vi "Convert RGB to HSL.vi"(11 "Color Box":u32(colorbox)=16777215) -> (1 "L (%)":dbl, 2 "S (%)":dbl, 3 "H (deg)":dbl format="%#_2p")   [LabVIEW 2015, in "ColorSelector.lvclass"]
doc: "This VI will convert the RGB Color Scale to the HSL Color Scale.\n<b> </b> <b> </b>\n©2017 Q Software Innovations, LLC (QSI)\nwritten by Quentin Alldredge\nproduced in LabVIEW 2015\n\nsupport@qsoftwareinnovations.com\nwww.qsoftwareinnovations.com\n\nAll rights reserved.\n\nRedistribution and use in source and binary forms, with or without modification, are permitted provided that the following conditions are met:\n\n * Redistributions of source code must retain the above copyright notice, this list of conditions and the following disclaimer.\n * Redistributions in binary form must reproduce the above copyright notice, this list of conditions and the following disclaimer in the documentation and/or other materials provided with the distribution.\n * Neither the name of Q Software Innovations, LLC. nor the names of its contributors may be used to endorse or promote products derived from this software without specific prior written permission.\n\nTHIS SOFTWARE IS PROVIDED BY THE COPYRIGHT HOLDERS AND CONTRIBUTORS \"AS IS\" AND ANY EXPRESS OR IMPLIED WARRANTIES, INCLUDING, BUT NOT LIMITED TO, THE IMPLIED WARRANTIES OF MERCHANTABILITY AND FITNESS FOR A PARTICULAR PURPOSE ARE DISCLAIMED. IN NO EVENT SHALL THE COPYRIGHT OWNER OR CONTRIBUTORS BE LIABLE FOR ANY DIRECT, INDIRECT, INCIDENTAL, SPECIAL, EXEMPLARY, OR CONSEQUENTIAL DAMAGES (INCLUDING, BUT NOT LIMITED TO, PROCUREMENT OF SUBSTITUTE GOODS OR SERVICES; LOSS OF USE, DATA, OR PROFITS; OR BUSINESS INTERRUPTION) HOWEVER CAUSED AND ON ANY THEORY OF LIABILITY, WHETHER IN CONTRACT, STRICT LIABILITY, OR TORT (INCLUDING NEGLIGENCE OR OTHERWISE) ARISING IN ANY WAY OUT OF THE USE OF THIS SOFTWARE, EVEN IF ADVISED OF THE POSSIBILITY OF SUCH DAMAGE."
uses:
  ColorSelector.lvclass
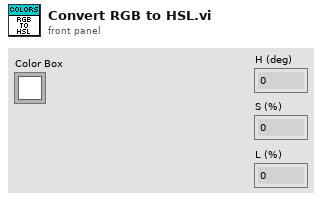
[diagram p1: front panel]
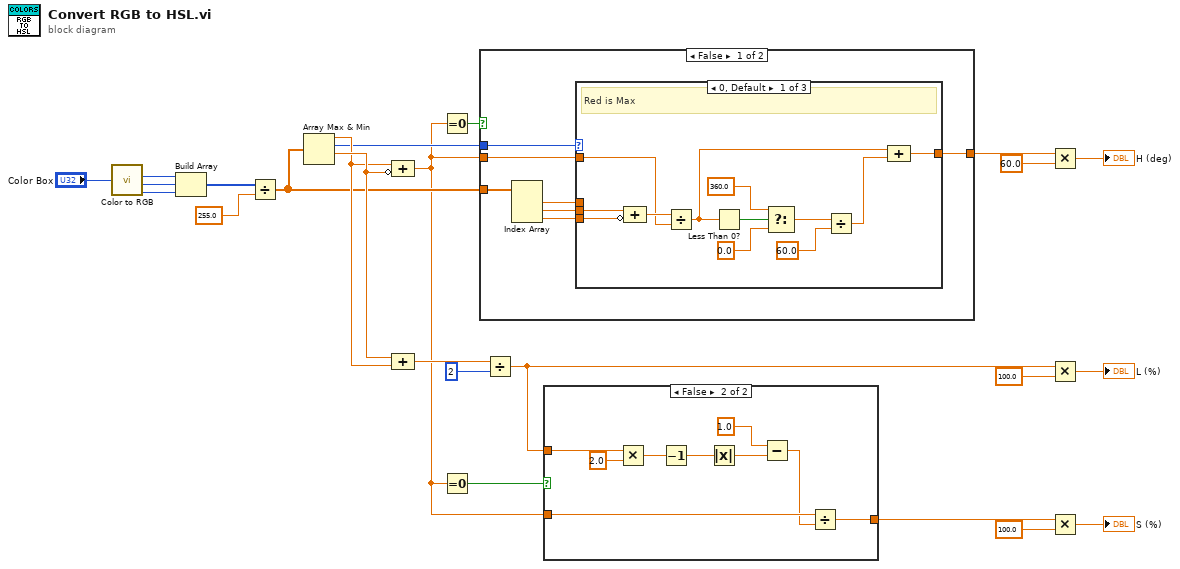
[diagram p0: block diagram]
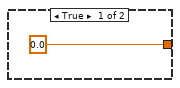
[diagram p2: hidden frame]
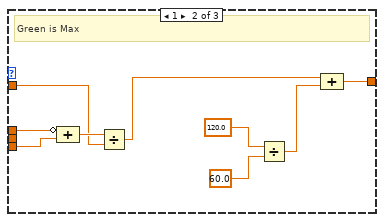
[diagram p3: hidden frame]
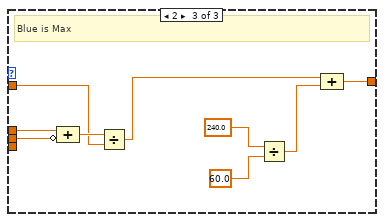
[diagram p4: hidden frame]
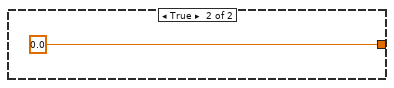
[diagram p5: hidden frame]
diagram:
  n1 = call <vilib>:"Color to RGB.vi"("Color"="Color Box") -> ("R"=w5:u8, "G"=w4:u8, "B"=w3:u8)  [unwired: 1 out]
  n2 = Build Array(w5, w4, w3) -> (w17:u8[])
  n3 = Divide(x=w17, y=255.0 ("x")) -> (x/y=w15:dbl[])
  n4 = Array Max & Min(array=w15) -> (max value=w22:dbl, max index (indices)=w19:i32, min value=w23:dbl)  [unwired: 1 out]
  n5 = Compound Arithmetic op=ADD(w22, invert w23) -> (w1:dbl)
  n6 = Compound Arithmetic op=ADD(w23, w22) -> (w21:dbl)
  n7 = Equal To 0?(x=w1) -> (x = 0?=w2:bool)
  n8 = Equal To 0?(x=w1) -> (x = 0?=w18:bool)
  n9 = case shown="False" w2 {
    tunnel: [w30 0.0] -> w13
    tunnel: w19 -> [w31 _]
    tunnel: w15 -> [w29 _]
    tunnel: w1 -> [w25 _]
    frame False {
      n10 = Index Array(array=w29) -> (element #1=w28:dbl, element #2=w27:dbl, element #3=w26:dbl)  [unwired: 3 in]
      n11 = case shown="0, Default" w31 {
        tunnel: w25 -> [w42 w51 w60]
        tunnel: [w34 w47 w56] -> w30
        tunnel: w28 -> [_ w45 w54]
        tunnel: w27 -> [w33 _ w53]
        tunnel: w26 -> [w32 w44 _]
        frame 0, Default {
          # "Red is Max"
          n12 = Compound Arithmetic op=ADD(w33, invert w32) -> (w43:dbl)
          n13 = Divide(x=w43, y=w42) -> (x/y=w36:dbl)
          n14 = Less Than 0?(x=w36) -> (x < 0?=w41:bool)
          n15 = Select(t=360.0 ("x"), s=w41, f=0.0 ("x")) -> (s? t:f=w38:dbl)
          n16 = Divide(x=w38, y=60.0) -> (x/y=w35:dbl)
          n17 = Compound Arithmetic op=ADD(w36, w35) -> (w34:dbl)
        }
        frame 1 {
          # "Green is Max"
          n18 = Compound Arithmetic op=ADD(invert w45, w44) -> (w52:dbl)
          n19 = Divide(x=w52, y=w51) -> (x/y=w49:dbl)
          n20 = Divide(x=120.0, y=60.0) -> (x/y=w48:dbl)
          n21 = Compound Arithmetic op=ADD(w49, w48) -> (w47:dbl)
        }
        frame 2 {
          # "Blue is Max"
          n22 = Compound Arithmetic op=ADD(w54, invert w53) -> (w61:dbl)
          n23 = Divide(x=w61, y=w60) -> (x/y=w58:dbl)
          n24 = Divide(x=240.0, y=60.0) -> (x/y=w57:dbl)
          n25 = Compound Arithmetic op=ADD(w58, w57) -> (w56:dbl)
        }
      }
    }
    frame True {
    }
  }
  n26 = Divide(x=w21, y=u8 2) -> (x/y=w10:dbl)
  n27 = case shown="False" w18 {
    tunnel: [0.0 ("y") w64] -> w7
    tunnel: w1 -> [_ w72]
    tunnel: w10 -> [_ w71]
    frame True {
    }
    frame False {
      n28 = Multiply(x=w71, y=2.0) -> (x*y=w69:dbl)
      n29 = Decrement(x=w69) -> (x-1=w68:dbl)
      n30 = Absolute Value(x=w68) -> (abs(x)=w67:dbl)
      n31 = Subtract(x=1.0 ("y"), y=w67) -> (x-y=w65:dbl)
      n32 = Divide(x=w72, y=w65) -> (x/y=w64:dbl)
    }
  }
  n33 = Multiply(x=w13, y=60.0) -> (x*y=→"H (deg)":dbl)
  n34 = Multiply(x=w10, y=100.0) -> (x*y=→"L (%)":dbl)
  n35 = Multiply(x=w7, y=100.0) -> (x*y=→"S (%)":dbl)
